vi "Preview Private Data Control Icon.vi"(11 "Theme Color":u32(colorbox)=255) -> (3 "Icon Image Out":picture)   [LabVIEW 2015, in "QControl Creation Wizard.lvclass"]
doc: "<b> </b> <b> </b>\n©2016 Q Software Innovations, LLC (QSI)\nwritten by Quentin Alldredge\nproduced in LabVIEW 2015\n\nsupport@qsoftwareinnovations.com\nwww.qsoftwareinnovations.com\n\nAll rights reserved.\n\nRedistribution and use in source and binary forms, with or without modification, are permitted provided that the following conditions are met:\n\n * Redistributions of source code must retain the above copyright notice, this list of conditions and the following disclaimer.\n * Redistributions in binary form must reproduce the above copyright notice, this list of conditions and the following disclaimer in the documentation and/or other materials provided with the distribution.\n * Neither the name of Q Software Innovations, LLC. nor the names of its contributors may be used to endorse or promote products derived from this software without specific prior written permission.\n\nTHIS SOFTWARE IS PROVIDED BY THE COPYRIGHT HOLDERS AND CONTRIBUTORS \"AS IS\" AND ANY EXPRESS OR IMPLIED WARRANTIES, INCLUDING, BUT NOT LIMITED TO, THE IMPLIED WARRANTIES OF MERCHANTABILITY AND FITNESS FOR A PARTICULAR PURPOSE ARE DISCLAIMED. IN NO EVENT SHALL THE COPYRIGHT OWNER OR CONTRIBUTORS BE LIABLE FOR ANY DIRECT, INDIRECT, INCIDENTAL, SPECIAL, EXEMPLARY, OR CONSEQUENTIAL DAMAGES (INCLUDING, BUT NOT LIMITED TO, PROCUREMENT OF SUBSTITUTE GOODS OR SERVICES; LOSS OF USE, DATA, OR PROFITS; OR BUSINESS INTERRUPTION) HOWEVER CAUSED AND ON ANY THEORY OF LIABILITY, WHETHER IN CONTRACT, STRICT LIABILITY, OR TORT (INCLUDING NEGLIGENCE OR OTHERWISE) ARISING IN ANY WAY OUT OF THE USE OF THIS SOFTWARE, EVEN IF ADVISED OF THE POSSIBILITY OF SUCH DAMAGE."
uses:
  QControl Creation Wizard.lvclass
  <vilib>/picture/picture.llb/imagedata.ctl
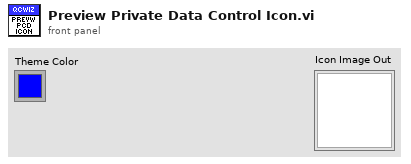
[diagram p1: front panel]
types:
  T1 = cluster{"left":i16, "top":i16, "right":i16, "bottom":i16}
  T2 = typedef "imagedata.ctl" = cluster{"image type":i32, "image depth":i32, "image":u8[], "mask":u8[], "colors":u32[], "Rectangle":cluster{"left":i16, "top":i16, "right":i16, "bottom":i16}}
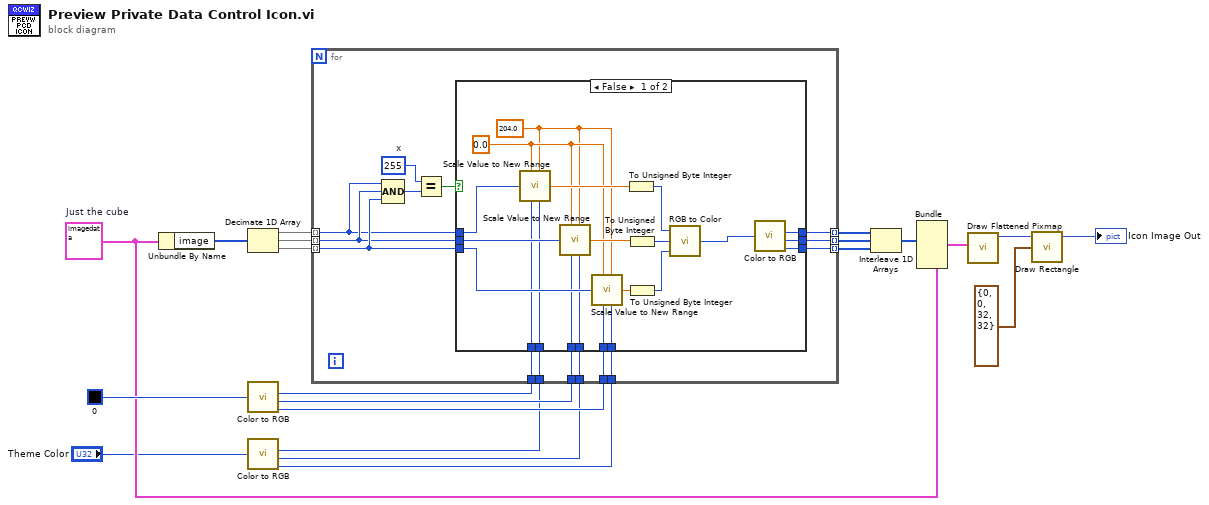
[diagram p0: block diagram]
diagram:
  w5 = T2 {"image type"=0, "image depth"=24, "image"=array[3072 elements], "mask"=[], "colors"=[], "Rectangle"={"left"=0, "top"=0, "right"=32, "bottom"=32}}  # Just the cube
  n1 = Unbundle By Name(w5) -> ("image"=w7:u8[])
  n2 = Decimate 1D Array(w7) -> (w14:u8[], w16:u8[], w15:u8[])
  n3 = call <vilib>:"Color to RGB.vi"("Color"=u32 0) -> ("R"=w10:u8, "G"=w12:u8, "B"=w21:u8)  [unwired: 1 out]
  n4 = call <vilib>:"Color to RGB.vi"("Color"="Theme Color") -> ("R"=w11:u8, "G"=w13:u8, "B"=w20:u8)  [unwired: 1 out]
  n5 = for {
    tunnel: w14 -> [w29] mode=indexing
    tunnel: w16 -> [w30] mode=indexing
    tunnel: w15 -> [w31] mode=indexing
    tunnel: w21 -> [w36]
    tunnel: w20 -> [w35]
    tunnel: [w34] -> w19 mode=indexing
    tunnel: [w33] -> w18 mode=indexing
    tunnel: [w32] -> w17 mode=indexing
    tunnel: w13 -> [w28]
    tunnel: w12 -> [w27]
    tunnel: w11 -> [w26]
    tunnel: w10 -> [w25]
    w23 = u8 255  # x
    n6 = Compound Arithmetic op=AND(w29, w30, w31) -> (w24:u8)
    n7 = Equal?(x=w23, y=w24) -> (x = y?=w22:bool)
    n8 = case shown="False" w22 {
      tunnel: w36 -> [w57 _]
      tunnel: w35 -> [w56 _]
      tunnel: [w55 w60] -> w34
      tunnel: [w54 w59] -> w33
      tunnel: [w53 w58] -> w32
      tunnel: w31 -> [w52 w58]
      tunnel: w30 -> [w51 w59]
      tunnel: w29 -> [w50 w60]
      tunnel: w28 -> [w49 _]
      tunnel: w27 -> [w48 _]
      tunnel: w26 -> [w47 _]
      tunnel: w25 -> [w46 _]
      frame False {
        w41 = 204.0 ("original maximum")
        w42 = 0.0 ("original minimum")
        n9 = call <vilib>:"Scale Value to New Range.vi"("original minimum"=w42, "original value"=w50, "new minimum"=w46, "original maximum"=w41, "new maximum"=w47) -> ("scaled value"=w45:dbl)  [unwired: 4 in]
        n10 = call <vilib>:"Scale Value to New Range.vi"("original minimum"=w42, "original value"=w51, "new minimum"=w48, "original maximum"=w41, "new maximum"=w49) -> ("scaled value"=w44:dbl)  [unwired: 4 in]
        n11 = call <vilib>:"Scale Value to New Range.vi"("original minimum"=w42, "original value"=w52, "new minimum"=w57, "original maximum"=w41, "new maximum"=w56) -> ("scaled value"=w43:dbl)  [unwired: 4 in]
        n12 = To Unsigned Byte Integer(number=w45) -> (unsigned 8bit integer=w40:u8)
        n13 = To Unsigned Byte Integer(number=w44) -> (unsigned 8bit integer=w39:u8)
        n14 = To Unsigned Byte Integer(number=w43) -> (unsigned 8bit integer=w38:u8)
        n15 = call <vilib>:"RGB to Color.vi"("B"=w38, "G"=w39, "R"=w40) -> ("Color"=w37:u32)
        n16 = call <vilib>:"Color to RGB.vi"("Color"=w37) -> ("R"=w55:u8, "G"=w54:u8, "B"=w53:u8)  [unwired: 1 out]
      }
      frame True {
      }
    }
  }
  n17 = Interleave 1D Arrays(w19, w18, w17) -> (w9:u8[])
  n18 = Bundle(cluster=w5, "image"=w9) -> (w6:T2)  [unwired: 5 in]
  n19 = call <vilib>:"Draw Flattened Pixmap.vi"("image data"=w6) -> ("new picture"=w4:picture)  [unwired: 8 in]
  n20 = call <vilib>:"Draw Rectangle.vi"("picture"=w4, "rect"=T1 {"left"=0, "top"=0, "right"=32, "bottom"=32}) -> ("new picture"=→"Icon Image Out":picture)  [unwired: 7 in]
